vi "Import Export - Dialog Get Masters and Slaves.vi"(8 "error in":errorcluster, 11 "Item Ref in":T1 format="%.0x") -> (0 "error out":errorcluster, 1 "EC Master Found?":bool, 2 "EC Master And Slaves":T2(array[cluster]), 3 "Item Ref out":T1 format="%.0x")   [LabVIEW 2017, in "Scan Engine Custom Device.lvlib"]
uses:
  Scan Engine Custom Device.lvlib
  <vilib>/NI Veristand/Custom Device API/Custom Device Item Ref.ctl
  Globals/Scan Engine GUIDs.vi
  <vilib>/NI Veristand/Custom Device Tools/Custom Device Utility Library/NI VeriStand - Search for All Items by GUID.vi
  <vilib>/NI Veristand/Custom Device Tools/Custom Device Utility Library/Custom Device Utility Library.lvlib
  <vilib>/NI Veristand/Custom Device API/Custom Device API.lvlib
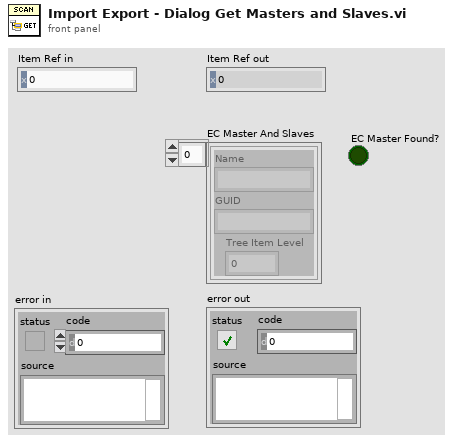
[diagram p1: front panel]
types:
  T1 = typedef "Custom Device API.lvlib/Custom Device Item Ref.ctl" = u64
  T2 = cluster{"Name":string, "GUID":string, "Tree Item Level":i32}[]
  T3 = typedef "Custom Device API.lvlib/Custom Device Item Info.ctl" = cluster{"Name":string, "Is Channel":bool, "GUID":string, "Is Waveform":bool}
  T4 = cluster{"Name":string, "GUID":string, "Tree Item Level":i32}
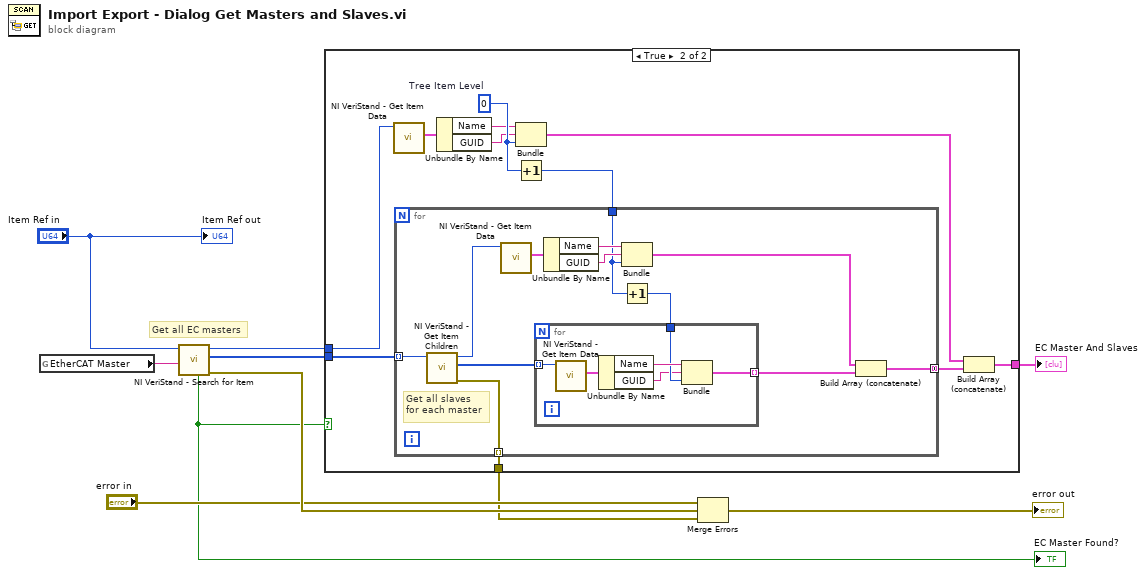
[diagram p0: block diagram]
diagram:
  # "Get all EC masters"
  n1 = global read "Scan Engine GUIDs.vi" "EtherCAT Master"() -> (w6:string)
  n2 = call-poly <vilib>:"NI VeriStand - Search for Item.vi"("Item GUID"=w6, "Section Ref in"="Item Ref in") -> ("error out"=w10:errorcluster, "Item Refs"=w7:T1[], "Section Ref out"=w8:T1, "Found"=w1:bool)  [unwired: 6 in]
  "EC Master Found?" <- w1
  n3 = case shown="True" w1 {
    tunnel: [_ w19] -> w9
    tunnel: w8 -> [_ w14]
    tunnel: w7 -> [_ w12]
    tunnel: [_ w11] -> w2
    frame False {
    }
    frame True {
      w21 = 0  # Tree Item Level
      n4 = call <vilib>:"NI VeriStand - Get Item Data.vi"("Item Ref in"=w14) -> ("Item Info"=w13:T3)  [unwired: 7 in, 3 out]
      n5 = Unbundle By Name(w13) -> ("Name"=w15:string, "GUID"=w20:string)
      n6 = Bundle("Name"=w15, "GUID"=w20, "Tree Item Level"=w21) -> (w16:T4)  [unwired: 1 in]
      n7 = Increment(x=w21) -> (x+1=w17:i32)
      n8 = for {
        tunnel: w12 -> [w32] mode=indexing
        tunnel: w17 -> [w23]
        tunnel: [w25] -> w18 mode=concatenating
        tunnel: [w22] -> w11 mode=indexing
        # "Get all slaves\nfor each master"
        n9 = call <vilib>:"NI VeriStand - Get Item Children.vi"("Item Ref in"=w32) -> ("error out"=w22:errorcluster, "Child Refs"=w33:T1[], "Item Ref out"=w29:T1)  [unwired: 7 in, 1 out]
        n10 = call <vilib>:"NI VeriStand - Get Item Data.vi"("Item Ref in"=w29) -> ("Item Info"=w30:T3)  [unwired: 7 in, 3 out]
        n11 = Unbundle By Name(w30) -> ("Name"=w31:string, "GUID"=w24:string)
        n12 = Bundle("Name"=w31, "GUID"=w24, w23) -> (w27:cluster{"Name":string, "GUID":string, i32})  [unwired: 1 in]
        n13 = Increment(x=w23) -> (x+1=w28:i32)
        n14 = for {
          tunnel: w33 -> [w37] mode=indexing
          tunnel: w28 -> [w35]
          tunnel: [w36] -> w26 mode=indexing
          n15 = call <vilib>:"NI VeriStand - Get Item Data.vi"("Item Ref in"=w37) -> ("Item Info"=w39:T3)  [unwired: 7 in, 3 out]
          n16 = Unbundle By Name(w39) -> ("Name"=w38:string, "GUID"=w34:string)
          n17 = Bundle("Name"=w38, "GUID"=w34, w35) -> (w36:cluster{"Name":string, "GUID":string, i32})  [unwired: 1 in]
        }
        n18 = Build Array (concatenate)(w27, w26) -> (w25:cluster{"Name":string, "GUID":string, i32}[])
      }
      n19 = Build Array (concatenate)(w16, w18) -> (w19:T2)
    }
  }
  "EC Master And Slaves" <- w9
  n20 = Merge Errors("error in", w10, w2) -> (→"error out":errorcluster)
  "Item Ref out" <- "Item Ref in"
